vi "sync_tasks.vi"() -> ()   [LabVIEW 2016, in "Utilities.lvlib" / "_TEST.lvlib"]
uses:
  <vilib>/DAQmx/write.llb/DAQmx Write (Analog Wfm 1Chan NSamp).vi
  <vilib>/DAQmx/create/channels.llb/DAQmx Create Channel (AO-Voltage-Basic).vi
  <vilib>/DAQmx/configure/timing.llb/DAQmx Timing (Sample Clock).vi
  <vilib>/DAQmx/miscellaneous.llb/DAQmx Fill In Error Info.vi
  <vilib>/Waveform/DWDTOps.llb/DWDT Analog to Digital.vi
  <vilib>/DAQmx/create/channels.llb/DAQmx Create Channel (CO-Pulse Generation-Time).vi
  <vilib>/DAQmx/configure/timing.llb/DAQmx Timing (Implicit).vi
  <vilib>/DAQmx/configure/trigger.llb/DAQmx Start Trigger (Digital Edge).vi
  _TEST.lvlib
  <vilib>/measure/NI_MABase.lvlib
  <vilib>/Analysis/NI_AALBase.lvlib
  <resource>/objmgr/daqmx.rc
panel:
  out "progress":dbl(slide) scale=0.0..1.0
  in  "repeats":i32=5
  in  "counter trigger (do)":tag="Dev1/ctr0"
  in  "delay line (ao)":tag="Dev1/ao0"
  out "scanning frequency (hz)":dbl
  out "sampling frequency (hz)":dbl
  out "daq output":T1(graph)
  out "generated position (v)":dbl[](array[numeric])
  out "generated position (ps)":dbl[](array[numeric])
  out "ideal position (v)":dbl[](array[numeric])
  in  "ratio (v/ps)":dbl=1.0
  in  "offset (ps)":dbl
  in  "range (ps)":dbl=5.0
  in  "# samples":i32=16
  in  "gate time (us)":dbl=200.0
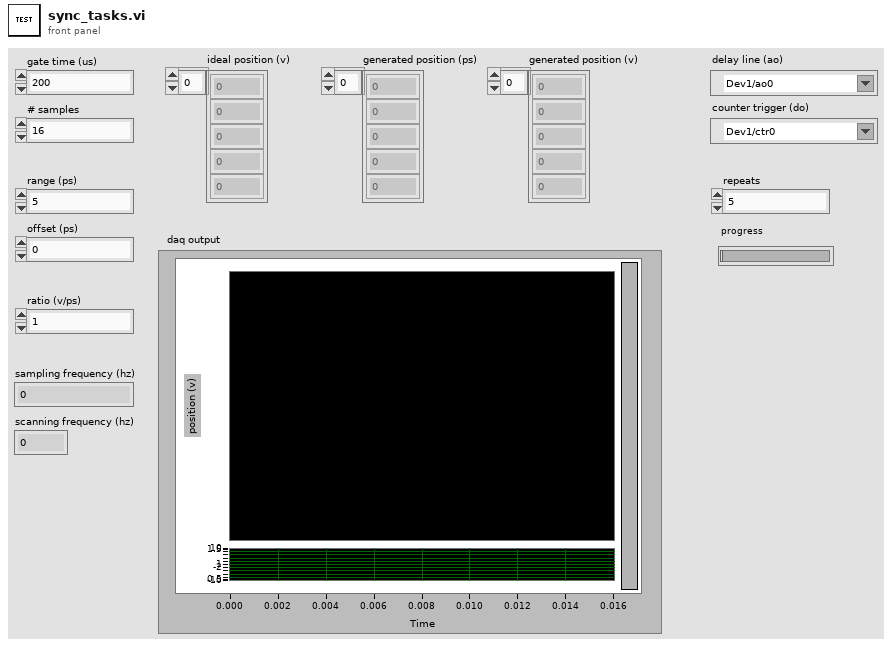
[diagram p1: front panel]
types:
  T1 = cluster{"signal out":waveform(dbl), "digital waveform":digitalwaveform}
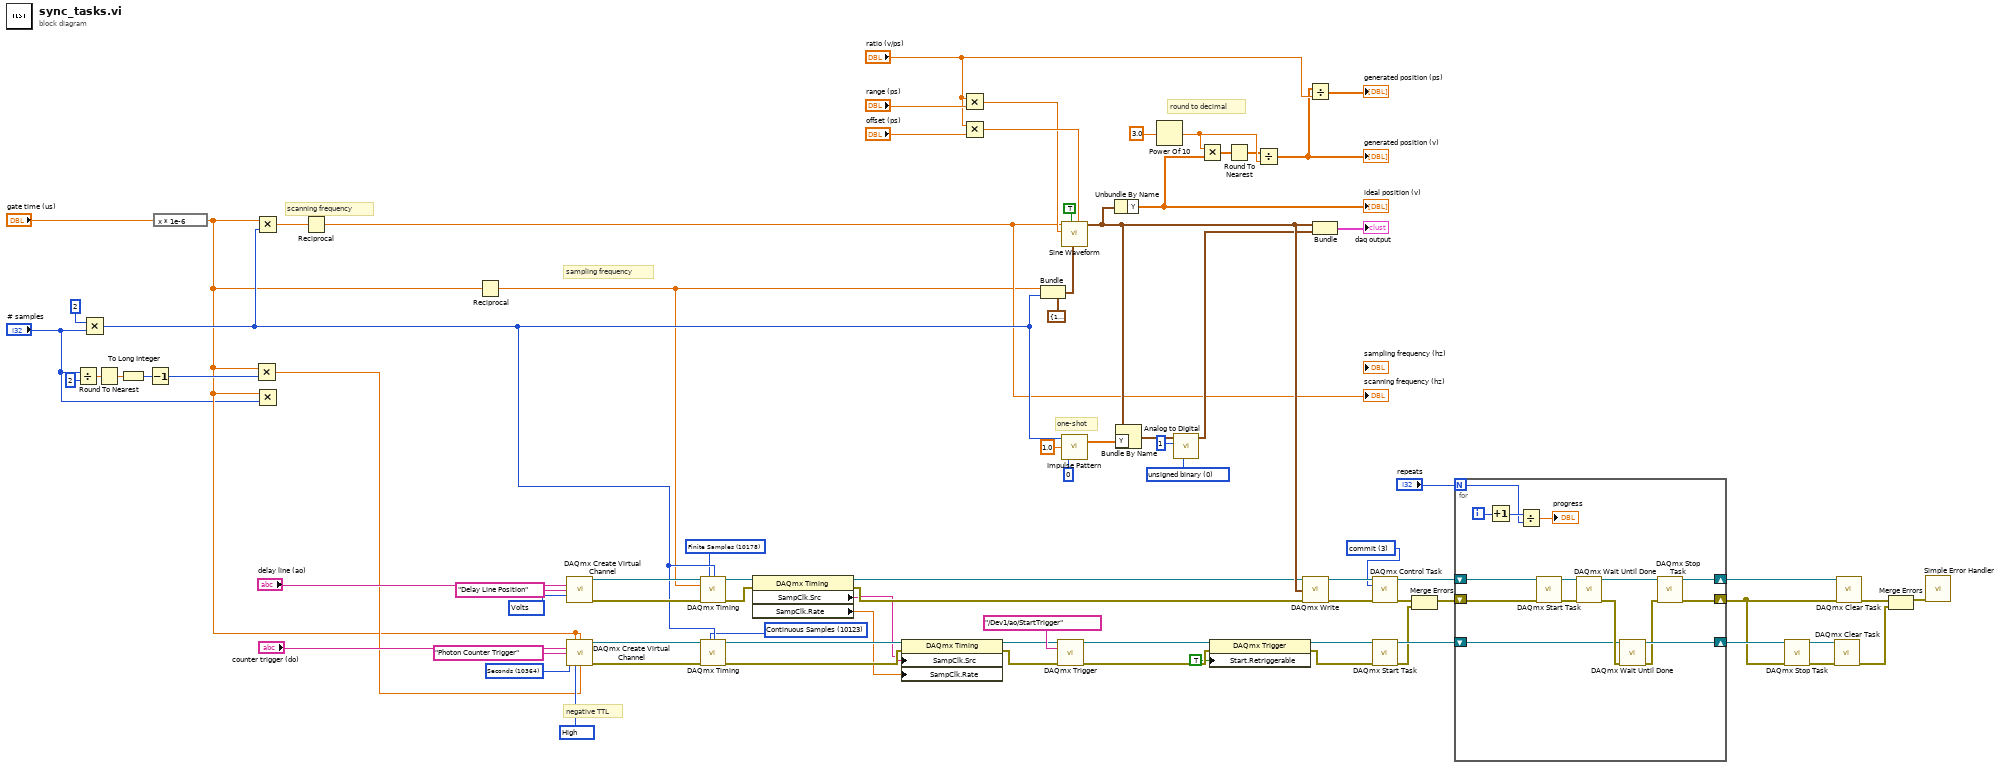
[diagram p0: block diagram]
diagram:
  w25 = 10123 items=["Finite Samples"=10178, "Continuous Samples"=10123, "Hardware Timed Single Point"=12522] ("sample mode")
  w15 = 3 items=["verify"=2, "reserve"=4, "commit"=3, "unreserve"=5, "abort"=6] ("action")
  w40 = 10364 items=["Seconds"=10364] ("units")
  w41 = 10192 items=["High"=10192, "Low"=10214] ("idle state")
  w26 = 10178 items=["Finite Samples"=10178, "Continuous Samples"=10123, "Hardware Timed Single Point"=12522] ("sample mode")
  w57 = 10348 items=["Volts"=10348, "From Custom Scale"=10065] ("units")
  w62 = u16 0 items=["unsigned binary", "offset binary", "2's complement"] ("data format (offset binary)")
  # "round to decimal"
  # "sampling frequency"
  # "scanning frequency"
  # "one-shot"
  # "negative TTL"
  n1 = Divide(x="# samples", y=2) -> (x/y=w6:dbl)
  n2 = Multiply(x=2, y="# samples") -> (x*y=w36:i32)
  n3 = Round To Nearest(number=w6) -> (nearest integer value=w3:dbl)
  n4 = To Long Integer(number=w3) -> (32bit integer=w2:i32)
  n5 = Decrement(x=w2) -> (x-1=w38:i32)
  n6 = expression code="x * 1e-6"("gate time (us)") -> (w27:dbl)
  n7 = Multiply(x=w27, y=w38) -> (x*y=w28:dbl)
  n8 = Multiply(x=w27, y=w36) -> (x*y=w78:dbl)
  n9 = Multiply(x=w27, y="# samples") -> ()  [unwired: 1 out]
  n10 = Reciprocal(x=w78) -> (1/x=w7:dbl)
  "scanning frequency (hz)" <- w7
  n11 = Reciprocal(x=w27) -> (1/x=w1:dbl)
  n12 = call-poly <vilib>:"DAQmx Create Virtual Channel.vi"("physical channels"="delay line (ao)", "name to assign"="Delay Line Position", "units"=w57) -> ("task out"=w56:refnum<k21>, "error out"=w53:errorcluster)  [unwired: 11 in]
  n13 = call-poly <vilib>:"DAQmx Create Virtual Channel.vi"("high time"=w27, "low time"=w27, "counter"="counter trigger (do)", "name to assign"="Photon Counter Trigger", "units"=w40, "idle state"=w41, "initial delay"=w28) -> ("task out"=w50:refnum<k21>, "error out"=w54:errorcluster)  [unwired: 7 in]
  n14 = call-poly <vilib>:"DAQmx Timing.vi"("task/channels in"=w56, "sample mode"=w26, "samples per channel"=w36, "rate"=w1, "error in"=w53) -> ("task out"=w42:refnum<k21>, "error out"=w23:errorcluster)  [unwired: 9 in]
  n15 = call-poly <vilib>:"DAQmx Timing.vi"("task/channels in"=w50, "sample mode"=w25, "samples per channel"=w36, "error in"=w54) -> ("task out"=w21:refnum<k21>, "error out"=w19:errorcluster)  [unwired: 10 in]
  n16 = property class="DAQmx Timing"(reference=w42, error in=w23) -> (reference out=w24:refnum<k21>, error out=w22:errorcluster, "SampClk.Src"=w17:tag, "SampClk.Rate"=w16:dbl)
  n17 = property class="DAQmx Timing"(reference=w21, error in=w19, "SampClk.Src"=w17, "SampClk.Rate"=w16) -> (reference out=w20:refnum<k21>, error out=w18:errorcluster)
  n18 = Multiply(x="ratio (v/ps)", y="range (ps)") -> (x*y=w79:dbl)
  n19 = Multiply(x="ratio (v/ps)", y="offset (ps)") -> (x*y=w80:dbl)
  n20 = Bundle(cluster=cluster{"Fs":dbl, "#s":dbl} {"Fs"=1000.0, "#s"=1000.0} ("sampling info"), "Fs"=w1, "#s"=w36) -> (w83:cluster{"Fs":dbl, "#s":dbl})
  n21 = call-poly <vilib>:"DAQmx Trigger.vi"("task/channels in"=w20, "source"=tag "/Dev1/ao/StartTrigger", "error in"=w18) -> ("task out"=w49:refnum<k21>, "error out"=w10:errorcluster)  [unwired: 11 in]
  n22 = call <vilib>:"Sine Waveform.vi"("offset"=w80, "sampling info"=w83, "reset signal"=TRUE, "amplitude"=w79, "frequency"=w7) -> ("signal out"=w51:waveform(dbl))  [unwired: 5 in, 1 out]
  n23 = call <vilib>:"Impulse Pattern.vi"("delay"=0, "amplitude"=1.0, "samples"=w36) -> ("Impulse Pattern"=w67:dbl[])  [unwired: 1 out]
  n24 = Unbundle By Name(w51) -> ("Y"=w74:dbl[])
  "ideal position (v)" <- w74
  n25 = Bundle By Name(cluster=w51, "Y"=w67) -> (w64:waveform(dbl))
  n26 = Power Of 10(x=3.0) -> (10^x=w70:dbl)
  n27 = call-poly <vilib>:"Analog to Digital.vi"("data format (offset binary)"=w62, "resolution (16 bit)"=1, "analog waveform"=w64) -> ("digital waveform"=w48:digitalwaveform)  [unwired: 5 in, 3 out]
  n28 = Multiply(x=w70, y=w74) -> (x*y=w69:dbl[])
  n29 = property class="DAQmx Trigger"(reference=w49, error in=w10, "Start.Retriggerable"=TRUE) -> (reference out=w11:refnum<k21>, error out=w9:errorcluster)
  n30 = Round To Nearest(number=w69) -> (nearest integer value=w68:dbl[])
  n31 = Divide(x=w68, y=w70) -> (x/y=w73:dbl[])
  "generated position (v)" <- w73
  n32 = call-poly <vilib>:"DAQmx Write.vi"("task/channels in"=w24, "data"=w51, "error in"=w22) -> ("task out"=w52:refnum<k21>, "error out"=w34:errorcluster)  [unwired: 10 in, 1 out]
  n33 = Divide(x=w73, y="ratio (v/ps)") -> (x/y=→"generated position (ps)":dbl[])
  n34 = Bundle("signal out"=w51, "digital waveform"=w48) -> (→"daq output":T1)  [unwired: 1 in]
  n35 = call <vilib>:"DAQmx Control Task.vi"("task/channels in"=w52, "action"=w15, "error in"=w34) -> ("task out"=w35:refnum<k21>, "error out"=w31:errorcluster)  [unwired: 11 in]
  n36 = call <vilib>:"DAQmx Start Task.vi"("task/channels in"=w11, "error in"=w9) -> ("task out"=w33:refnum<k21>, "error out"=w29:errorcluster)  [unwired: 12 in]
  n37 = Merge Errors(w31, w29) -> (w30:errorcluster)
  n38 = for {
    N: "repeats" -> [w88]
    shift-right: [w99] -> w46
    shift-left: w35 -> [w92]
    shift-right: [w96] -> w47
    shift-left: w33 -> [w85]
    shift-right: [w93] -> w13
    shift-left: w30 -> [w86]
    i -> [w90]
    n39 = Increment(x=w90) -> (x+1=w89:i32)
    n40 = Divide(x=w89, y=w88) -> (x/y=→"progress":dbl)
    n41 = call <vilib>:"DAQmx Start Task.vi"("task/channels in"=w92, "error in"=w86) -> ("task out"=w98:refnum<k21>, "error out"=w97:errorcluster)  [unwired: 12 in]
    n42 = call <vilib>:"DAQmx Wait Until Done.vi"("task/channels in"=w98, "error in"=w97) -> ("task out"=w94:refnum<k21>, "error out"=w91:errorcluster)  [unwired: 12 in]
    n43 = call <vilib>:"DAQmx Wait Until Done.vi"("task/channels in"=w85, "error in"=w91) -> ("task out"=w96:refnum<k21>, "error out"=w95:errorcluster)  [unwired: 12 in]
    n44 = call <vilib>:"DAQmx Stop Task.vi"("task/channels in"=w94, "error in"=w95) -> ("task out"=w99:refnum<k21>, "error out"=w93:errorcluster)  [unwired: 12 in]
  }
  n45 = call <vilib>:"DAQmx Stop Task.vi"("task/channels in"=w47, "error in"=w13) -> ("task out"=w14:refnum<k21>, "error out"=w12:errorcluster)  [unwired: 12 in]
  n46 = call <vilib>:"DAQmx Clear Task.vi"("task in"=w14, "error in"=w12) -> ("error out"=w44:errorcluster)  [unwired: 13 in]
  n47 = call <vilib>:"DAQmx Clear Task.vi"("task in"=w46, "error in"=w13) -> ("error out"=w45:errorcluster)  [unwired: 13 in]
  n48 = Merge Errors(w45, w44) -> (w43:errorcluster)
  n49 = call <vilib>:"Simple Error Handler.vi"("error in (no error)"=w43) -> ()  [unwired: 4 in, 5 out]
